vi "Path to Example Theme--constant.vi"() -> (3 "Path to Example Theme":path)   [LabVIEW 2021]
doc: "CONSTANT VI - defines the user VI tag for the theme mode\n\n<b>Code Developed By:</b>\nDaniel Coons\nTechnology Service Corporation\nwww.tsc.com/atcs"
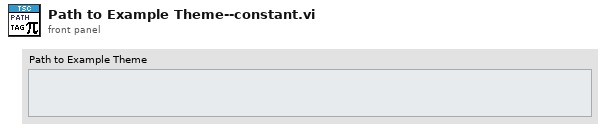
[diagram p1: front panel]
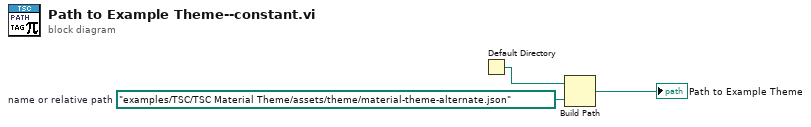
[diagram p0: block diagram]
diagram:
  w3 = path "examples/TSC/TSC Material Theme/assets/theme/material-theme-alternate.json"  # name or relative path
  n1 = Default Directory() -> (w1:path)
  n2 = Build Path(base path=w1, name or relative path=w3) -> (appended path=→"Path to Example Theme":path)
